vi "Log_Data.vi"(8 "error in (no error)":errorcluster, 10 "Data":sgl[][](array[numeric]), 11 "Logger_Data In":T1) -> (0 "error out":errorcluster, 3 "Logger_Data Out":T1)   [LabVIEW 2019, in "Data_Logger.lvlib"]
uses:
  Data_Logger.lvlib
  Logger_Data.ctl
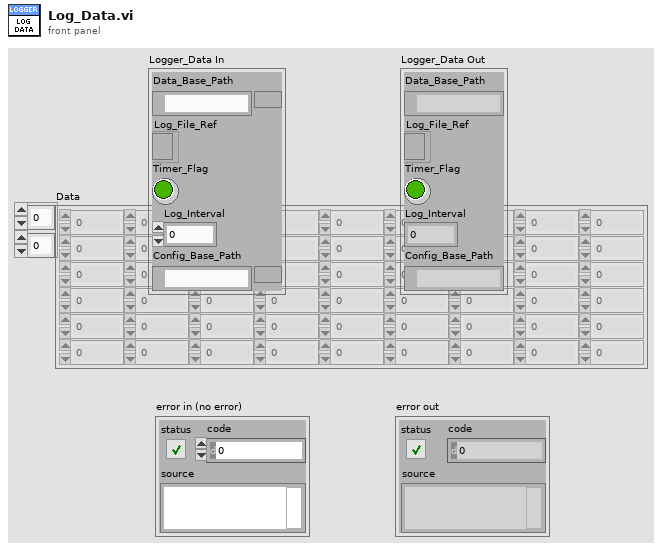
[diagram p1: front panel]
types:
  T1 = typedef "Data_Logger.lvlib/Logger_Data.ctl" = cluster{"Data_Base_Path":path, "Log_File_Ref":refnum<file>, "Timer_Flag":bool, "Log_Interval":dbl, "Config_Base_Path":path}
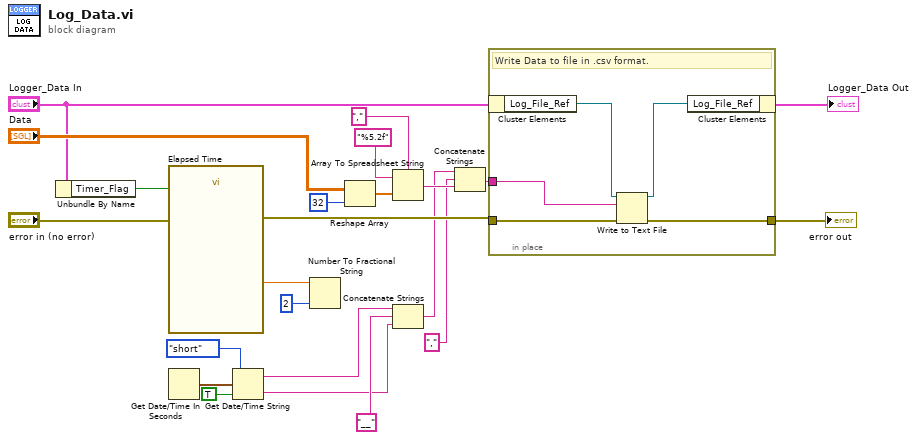
[diagram p0: block diagram]
diagram:
  n1 = Unbundle By Name("Logger_Data In") -> ("Timer_Flag"=w8:bool)
  n2 = call "Elapsed Time"("Reset"=w8, "error in (no error)"="error in (no error)") -> ("Elapsed Time (s)"=w11:dbl, "error out"=w15:errorcluster)  [unwired: 10 in, 6 out]
  n3 = Get Date/Time In Seconds() -> (seconds since 1Jan1904=w7:timestamp)
  n4 = Get Date/Time String(date format (0)=enum16{"short", "long", "abbreviated"}."short", seconds (now)=w7, want seconds? (F)=TRUE) -> (date string=w3:string, time string=w2:string)
  n5 = Number To Fractional String(number=w11, precision (6)=i16 2) -> ()  [unwired: 2 in, 1 out]
  n6 = Reshape Array("Data", 32 ("dimension size")) -> (w19:sgl[])
  n7 = Array To Spreadsheet String(delimiter (Tab)=",", array=w19, 3:"%5.2f" ("format string")) -> (spreadsheet string=w13:string)
  n8 = Concatenate Strings(w3, "__", w2) -> (w1:string)
  n9 = Concatenate Strings(w1, "," ("string"), w13) -> (w14:string)
  n10 = in-place {
    in-place-border: w15 -> [w26]
    in-place-border: [w25] -> w22
    in-place-border: w14 -> [w24]
    # "Write Data to file in .csv format."
    n11 = in-place-cluster #1("Logger_Data In") -> ("Log_File_Ref"=w28:refnum<file>)
    n12 = Write to Text File(file (use dialog)=w28, text=w24, error in=w26) -> (refnum out=w27:refnum<file>, error out=w25:errorcluster)  [unwired: 1 in, 1 out]
    n13 = in-place-cluster #1("Log_File_Ref"=w27) -> (→"Logger_Data Out":T1)
  }
  "error out" <- w22
